vi "Get UUID.vi"(7 "remove hyphen (F)":bool, 8 "error in (no error)":errorcluster) -> (0 "error out":errorcluster, 2 "found?":bool, 3 "CSP UUID":string)   [LabVIEW 2013]
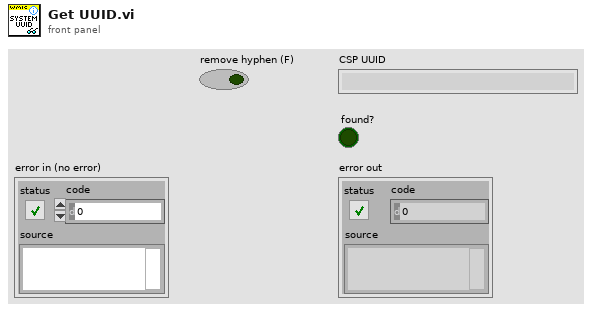
[diagram p1: front panel]
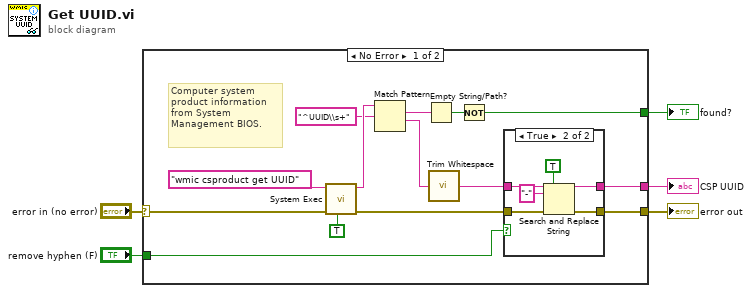
[diagram p0: block diagram]
diagram:
  n1 = case shown="No Error" "error in (no error)" {
    selector: "error in (no error)" -> [w11 w28]
    tunnel: [w9 _] -> w5
    tunnel: [w12 _] -> w4
    tunnel: [w7 w28] -> w3
    tunnel: "remove hyphen (F)" -> [w6 _]
    frame No Error {
      # "Computer system product information from System Management BIOS."
      n2 = call <vilib>:"System Exec.vi"("run minimized? (F)"=TRUE, "error in (no error)"=w11, "command line"="wmic csproduct get UUID") -> ("error out"=w8:errorcluster, "standard output"=w17:string)  [unwired: 5 in, 2 out]
      n3 = Match Pattern(string=w17, regular expression="^UUID\\s+") -> (match substring=w14:string, after substring=w15:string)  [unwired: 1 in, 2 out]
      n4 = Empty String/Path?(string/path=w14) -> (empty?=w13:bool)
      n5 = call <vilib>:"Trim Whitespace.vi"("string"=w15) -> ("trimmed string"=w10:string)  [unwired: 1 in]
      n6 = Not(x=w13) -> (.not. x?=w12:bool)
      n7 = case shown="True" w6 {
        tunnel: w10 -> [w21 w27]
        tunnel: [w21 w26] -> w9
        tunnel: w8 -> [w20 w25]
        tunnel: [w20 w24] -> w7
        frame False {
        }
        frame True {
          n8 = Search and Replace String(replace all?=TRUE ("replace all? (F)"), input string=w27, search string="-", error in=w25) -> (result string=w26:string, error out=w24:errorcluster)  [unwired: 4 in, 2 out]
        }
      }
    }
    frame Error {
    }
  }
  "CSP UUID" <- w5
  "found?" <- w4
  "error out" <- w3
